vi "Set Manual Timebase.vi"(8 "error in (no error)":errorcluster, 9 "Timebase":dbl, 11 "MSOX6004 in":refnum<class "MSOX6004.lvclass">) -> (0 "error out":errorcluster, 3 "MSOX6004 out":refnum<class "MSOX6004.lvclass">)   [LabVIEW 2018, in "MSOX6004.lvlib" / "MSOX6004.lvclass"]
uses:
  MSOX6004.lvclass
  MSOX6004.lvclass/MSOX6004.ctl
  <instrlib>/Keysight InfiniiVision/Keysight InfiniiVision.lvlib
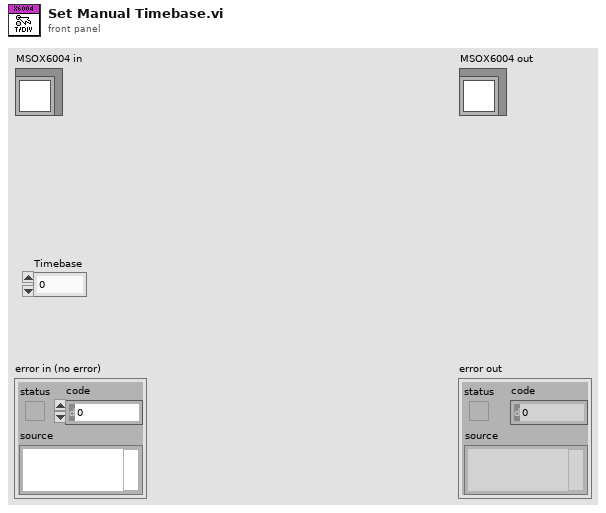
[diagram p1: front panel]
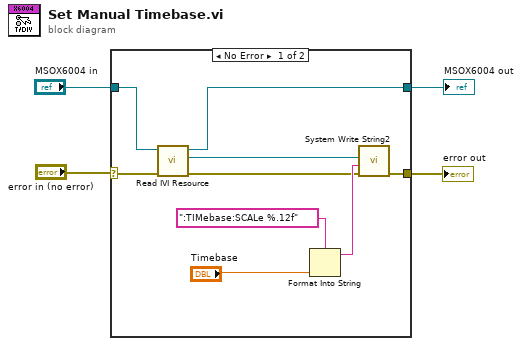
[diagram p0: block diagram]
diagram:
  n1 = case shown="No Error" "error in (no error)" {
    selector: "error in (no error)" -> [w13 w15]
    tunnel: [w8 w15] -> w1
    tunnel: [w11 w14] -> w4
    tunnel: "MSOX6004 in" -> [w12 w14]
    frame No Error {
      n2 = call "Read IVI Resource.vi"("error in (no error)"=w13, "MSOX6004 in"=w12) -> ("error out"=w5:errorcluster, "IVI Resource"=w6:refnum<k15>, "MSOX6004 out"=w11:refnum<class "MSOX6004.lvclass">)  [unwired: 7 in]
      n3 = Format Into String(format string=":TIMebase:SCALe %.12f", "Timebase") -> (resulting string=w9:string)  [unwired: 2 in, 1 out]
      n4 = call <instrlib>:"System Write String2.vi"("error in (no error)"=w5, "Data"=w9, "instrument handle"=w6) -> ("error out"=w8:errorcluster)  [unwired: 7 in, 1 out]
    }
    frame Error {
    }
  }
  "error out" <- w1
  "MSOX6004 out" <- w4
